vi "MListbox Check Test Result.vi"(8 "error in (no error)":errorcluster, 10 "Column Inex":u16=4, 11 "Multicolumn ListBox in":refnum<class "Multicolumn ListBox.lvclass">) -> (0 "error out":errorcluster, 2 "Pass?":bool, 3 "Multicolumn ListBox out":refnum<class "Multicolumn ListBox.lvclass">)   [LabVIEW 2012, in "Multicolumn ListBox.lvclass"]
uses:
  Multicolumn ListBox.lvclass
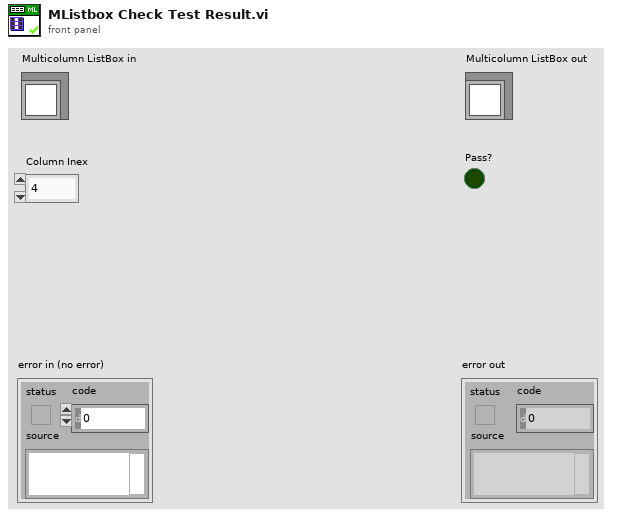
[diagram p1: front panel]
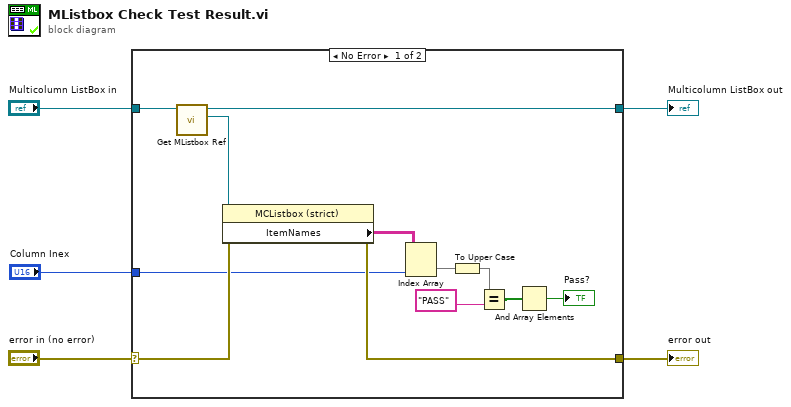
[diagram p0: block diagram]
diagram:
  n1 = case shown="No Error" "error in (no error)" {
    selector: "error in (no error)" -> [w15 w19]
    tunnel: [w13 w19] -> w4
    tunnel: [w14 w18] -> w2
    tunnel: "Multicolumn ListBox in" -> [w17 w18]
    tunnel: "Column Inex" -> [w11 _]
    frame No Error {
      n2 = call "Get MListbox Ref.vi"("Multicolumn ListBox in"=w17) -> ("MListbox Ref"=w16:refnum<vi>, "Multicolumn ListBox out"=w14:refnum<class "Multicolumn ListBox.lvclass">)  [unwired: 8 in, 1 out]
      n3 = property class="MCListbox (strict)"(reference=w16, error in=w15) -> (error out=w13:errorcluster, "ItemNames"=w12:string[][])  [unwired: 1 out]
      n4 = Index Array(array=w12, index (col)=w11) -> (element=w10:string[])  [unwired: 1 in]
      n5 = To Upper Case(1:w10) -> (0:w9:string[])
      n6 = Equal?(x=w9, y="PASS") -> (x = y?=w7:bool[])
      n7 = And Array Elements(Boolean array=w7) -> (logical AND=→"Pass?":bool)
    }
    frame Error {
    }
  }
  "error out" <- w4
  "Multicolumn ListBox out" <- w2
